vi "IniToken Load From LabVIEW.ini.vi"(8 "error in (no error)":errorcluster, 11 "IniTokenCluster":T1) -> (0 "error out":errorcluster, 3 "Cluster":T2)   [LabVIEW 2020]
uses:
  Def-IniTokenCluster.ctl
  <resource>/dialog/lvconfig.llb/LV Config Read String.vi
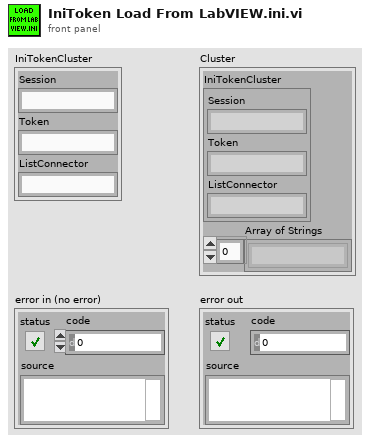
[diagram p1: front panel]
types:
  T1 = typedef "Def-IniTokenCluster.ctl" = cluster{"Session":string, "Token":string, "ListConnector":string}
  T2 = cluster{"IniTokenCluster":T1, "Array of Strings":string[]}
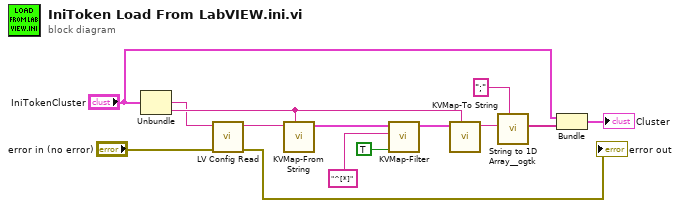
[diagram p0: block diagram]
diagram:
  n1 = Unbundle("IniTokenCluster") -> ("Token"=w7:string, "ListConnector"=w8:string)  [unwired: 1 out]
  n2 = call-poly <resource>:"LV Config Read.vi"("error in"="error in (no error)", "key"=w7) -> ("error out"=→"error out":errorcluster, "value"=w1:string)  [unwired: 3 in, 1 out]
  n3 = call "KVMap-From String.vi"("delimiter (Tab)"=w8, "value"=w1) -> ("Cluster"=w2:cluster{string[], string[]})  [unwired: 9 in]
  n4 = call "KVMap-Filter.vi"("T->First/F->Second(F)"=TRUE, "filter"="^[*]", "Cluster in"=w2) -> ("Cluster out"=w3:cluster{string[], string[]})  [unwired: 8 in]
  n5 = call "KVMap-To String.vi"("string"=w8, "Cluster"=w3) -> ("value"=w6:string)  [unwired: 9 in]
  n6 = call <userlib>:"String to 1D Array__ogtk.vi"("delimiter (Tab)"=";", "string"=w6) -> ("Array of Strings"=w10:string[])  [unwired: 9 in]
  n7 = Bundle("IniTokenCluster"="IniTokenCluster", "Array of Strings"=w10) -> (→"Cluster":T2)  [unwired: 1 in]
